vi "gaussmeter_measure.vi"(8 "error in (no error)":errorcluster, 10 "Switch Gaussmeter":bool, 11 "VISA resource name":refnum<visa-resource-name>) -> (0 "error out":errorcluster, 1 "Field Range":u16(ring)=1 items=["1 - Lowest"=1, "2"=2, "3"=3, "4 - Highest"=4], 2 "Field Reading":dbl format="%^.3e", 3 "VISA resource name out":refnum<visa-resource-name>, 4 "Field Units":u16(ring)=1 items=["Gauss"=1, "Tesla"=2, "Oersted"=3, "Amp/Meter"=4])   [LabVIEW 2016]
uses:
  <instrlib>/Lake Shore 425/Public/Data/Field Data (Single Reading).vi
  <instrlib>/Lake Shore 425/Lake Shore 425.lvlib
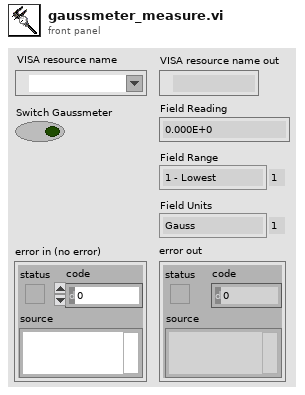
[diagram p1: front panel]
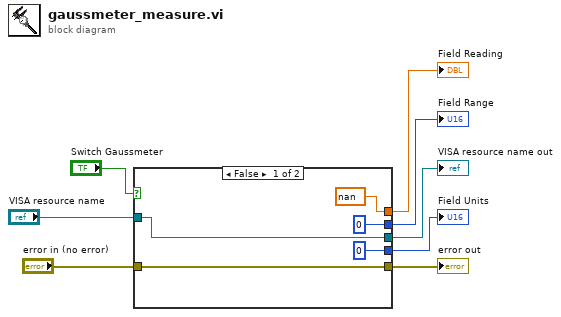
[diagram p0: block diagram]
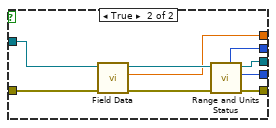
[diagram p2: hidden frame]
diagram:
  n1 = case shown="False" "Switch Gaussmeter" {
    tunnel: "VISA resource name" -> [w13 w21]
    tunnel: "error in (no error)" -> [w12 w20]
    tunnel: [w13 w19] -> w6
    tunnel: [u16 0 ("Field Range") w18] -> w5
    tunnel: [u16 0 ("Field Units") w17] -> w4
    tunnel: [nan ("Field Reading") w16] -> w3
    tunnel: [w12 w14] -> w2
    frame False {
    }
    frame True {
      n2 = call-poly <instrlib>:"Field Data.vi"("error in (no error)"=w20, "VISA resource name"=w21) -> ("error out"=w15:errorcluster, "Field Reading"=w16:dbl, "VISA resource name out"=w22:refnum<visa-resource-name>)  [unwired: 7 in]
      n3 = call <instrlib>:"Range and Units Status.vi"("error in (no error)"=w15, "VISA resource name"=w22) -> ("error out"=w14:errorcluster, "Field Units"=w17:u16, "VISA resource name out"=w19:refnum<visa-resource-name>, "Field Range"=w18:u16)  [unwired: 5 in, 1 out]
    }
  }
  "VISA resource name out" <- w6
  "Field Range" <- w5
  "Field Units" <- w4
  "Field Reading" <- w3
  "error out" <- w2
